vi "bgk_3475_protocol.vi"(11 "read from buffer":string) -> (3 "data":sgl caption="数据")   [LabVIEW 2015]
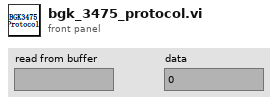
[diagram p1: front panel]
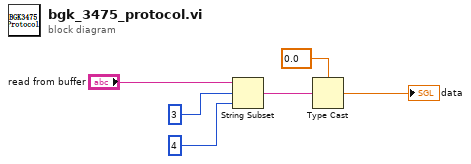
[diagram p0: block diagram]
diagram:
  n1 = String Subset(string="read from buffer", offset (0)=3 ("偏移量(0)"), length (rest)=4 ("长度（剩余）")) -> (substring=w4:string)
  n2 = Type Cast(type=sgl 0.0, x=w4) -> (*(type *) &x=→"data":sgl)
